vi "Choreo_TrajectoryState_Interpolate.vi"(9 "T":dbl, 10 "EndValue TrajectoryState":T1, 11 "ChoreoTrajectoryState":T1) -> (3 "Interpolated ChoreoTrajectoryState":T1)   [LabVIEW 2019]
doc: "Interpolate between two trajectory states.\n\nInputs:\n - ChoreoTrajectoryState - cluster - The earlier trajectory state.\n - EndValue_TrajectoryState - cluster - The next state. It should have a timestamp after this state.\n - T - double - the timestamp of the interpolated state. It should be between this state and endValue.\n\nOutputs:\n - InterpolatedState - cluster - Interpolated trajectory state."
uses:
  TypeDef/ChoreoTrajectoryState.ctl
  <vilib>/Rock Robotics/WPI/ThirdParty/JAS_Junk/TrajLib/Twist2d_GetAll.vi
  <vilib>/Rock Robotics/WPI/ThirdParty/JAS_Junk/TrajLib/Twist2d_Create.vi
  <vilib>/Rock Robotics/WPI/ThirdParty/JAS_Junk/TrajLib/Pose2d_New.vi
  <vilib>/Rock Robotics/WPI/ThirdParty/JAS_Junk/TrajLib/MathUtil_Clamp.vi
  <vilib>/Rock Robotics/WPI/ThirdParty/JAS_Junk/TrajLib/Rotation2d_CreateAngle.vi
  <vilib>/Rock Robotics/WPI/ThirdParty/JAS_Junk/TrajLib/Translation2d_Create.vi
  <vilib>/Rock Robotics/WPI/ThirdParty/JAS_Junk/TrajLib/Pose2d_Log.vi
  <vilib>/Rock Robotics/WPI/ThirdParty/JAS_Junk/TrajLib/Pose2d_Exp.vi
  <vilib>/Rock Robotics/WPI/ThirdParty/JAS_Junk/TrajLib/Trajectory_Library.lvlib
  ChoreoLib.lvlib
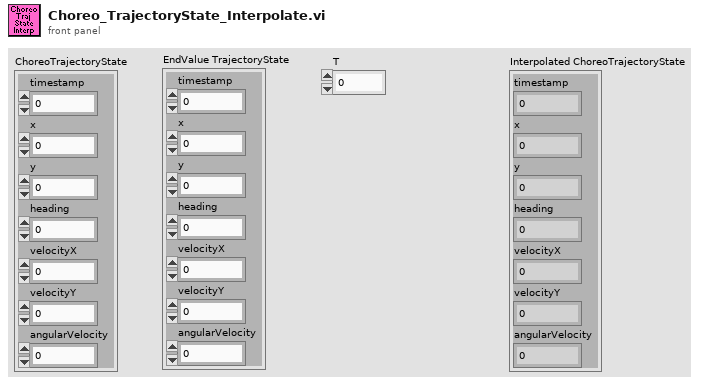
[diagram p1: front panel]
types:
  T1 = typedef "ChoreoLib.lvlib/ChoreoTrajectoryState.ctl" = cluster{"timestamp":dbl, "x":dbl, "y":dbl, "heading":dbl, "velocityX":dbl, "velocityY":dbl, "angularVelocity":dbl}
  T2 = typedef "Trajectory_Library.lvlib/POSE2D.ctl" = cluster{"TRANSLATION":T3, "ROTATION":T4}
  T3 = typedef "Trajectory_Library.lvlib/TRANSLATION2D.ctl" = cluster{"X":dbl, "Y":dbl}
  T4 = typedef "Trajectory_Library.lvlib/ROTATION2D.ctl" = cluster{"VALUE":dbl, "COS":dbl, "SIN":dbl}
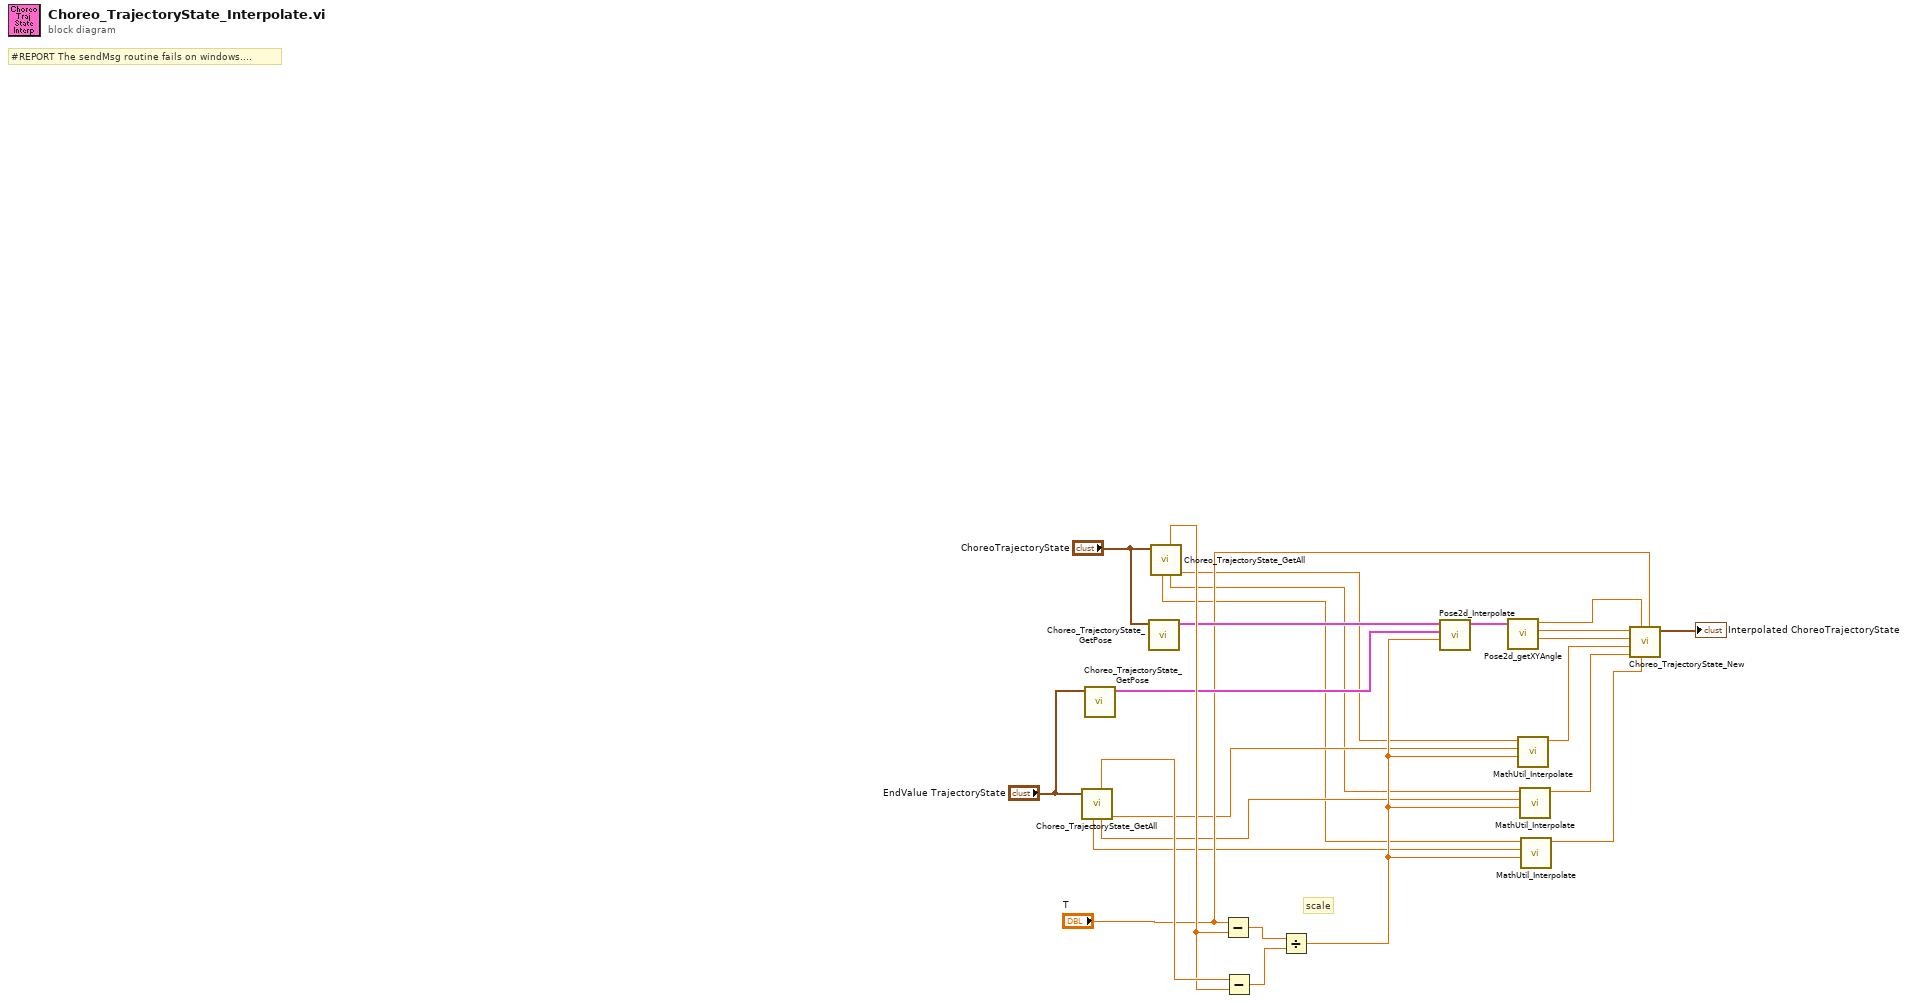
[diagram p0: block diagram]
diagram:
  # "scale"
  # "#REPORT The sendMsg routine fails on windows...."
  n1 = call "Choreo_TrajectoryState_GetAll.vi"("ChoreoTrajectoryState"="EndValue TrajectoryState") -> ("velocityX"=w8:dbl, "velocityY"=w6:dbl, "timestamp"=w23:dbl, "angularVelocity"=w4:dbl)  [unwired: 4 in, 3 out]
  n2 = call "Choreo_TrajectoryState_GetPose.vi"("ChoreoTrajectoryState"="EndValue TrajectoryState") -> ("POSE2D"=w16:T2)  [unwired: 10 in]
  n3 = call "Choreo_TrajectoryState_GetPose.vi"("ChoreoTrajectoryState"="ChoreoTrajectoryState") -> ("POSE2D"=w17:T2)  [unwired: 10 in]
  n4 = call "Choreo_TrajectoryState_GetAll.vi"("ChoreoTrajectoryState"="ChoreoTrajectoryState") -> ("velocityX"=w9:dbl, "velocityY"=w7:dbl, "timestamp"=w22:dbl, "angularVelocity"=w5:dbl)  [unwired: 4 in, 3 out]
  n5 = Subtract(x="T", y=w22) -> (x-y=w21:dbl)
  n6 = Subtract(x=w23, y=w22) -> (x-y=w20:dbl)
  n7 = Divide(x=w21, y=w20) -> (x/y=w10:dbl)
  n8 = call <vilib>:"Pose2d_Interpolate.vi"("T"=w10, "EndValue Pose"=w16, "in POSE"=w17) -> ("Interpolated Pose"=w15:T2)  [unwired: 8 in]
  n9 = call <vilib>:"Pose2d_getXYAngle.vi"("in POSE"=w15) -> ("Angle"=w11:dbl, "Y"=w12:dbl, "X"=w13:dbl)  [unwired: 8 in]
  n10 = call <vilib>:"MathUtil_Interpolate.vi"("T"=w10, "EndValue"=w8, "StartValue"=w9) -> ("InterpolatedValue"=w3:dbl)  [unwired: 8 in]
  n11 = call <vilib>:"MathUtil_Interpolate.vi"("T"=w10, "EndValue"=w6, "StartValue"=w7) -> ("InterpolatedValue"=w2:dbl)  [unwired: 8 in]
  n12 = call <vilib>:"MathUtil_Interpolate.vi"("T"=w10, "EndValue"=w4, "StartValue"=w5) -> ("InterpolatedValue"=w1:dbl)  [unwired: 8 in]
  n13 = call "Choreo_TrajectoryState_New.vi"("timestamp"="T", "angularVelocity"=w1, "x"=w13, "velocityY"=w2, "velocityX"=w3, "heading"=w11, "y"=w12) -> ("ChoreoTrajectoryState"=→"Interpolated ChoreoTrajectoryState":T1)  [unwired: 4 in]
